vi "5-1 velocità intervento.vi"(2 "stop":bool) -> (0 "delay":u32, 1 "time":u32, 3 "ALARM":bool)   [LabVIEW 2012]
panel:
  # "Realizzare un VI capace di misurare la velocità di intervento di un operatore\n\nValutare il tempo di risposta (Delay) che intercorre tra l'accensione dell'allarme  \ne la pressione del tasto stop e il tempo (Time) di esecuzione del VI."
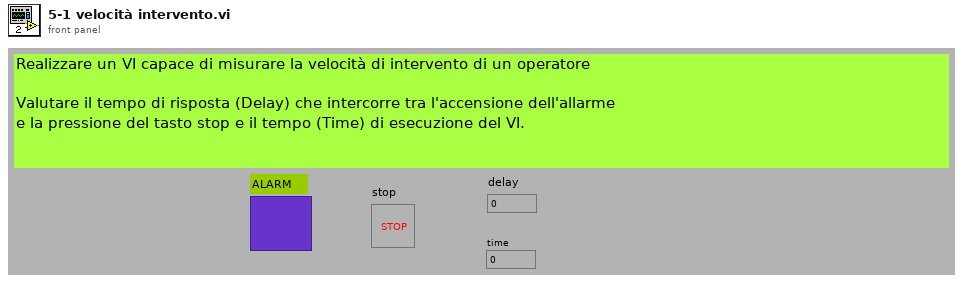
[diagram p1: front panel]
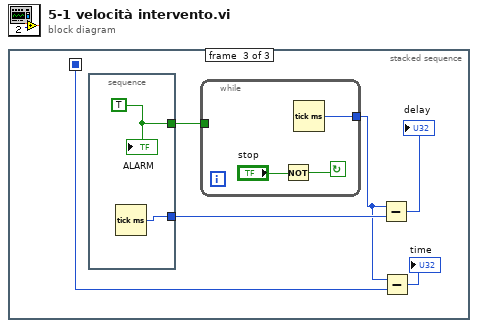
[diagram p0: block diagram]
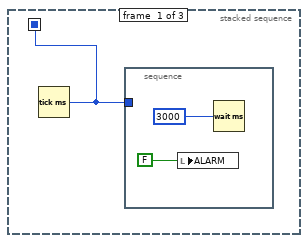
[diagram p2: hidden frame]
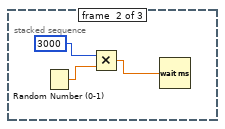
[diagram p3: hidden frame]
diagram:
  n1 = stacked-sequence {
    seq-local: [w1 _ _] -> [_ _ w9]
    frame #0 {
      n2 = Tick Count (ms)() -> (millisecond timer value=w1:u32)
      n3 = stacked-sequence {
        tunnel: w1 -> [_]
        frame #0 {
          n4 = local write "ALARM"(FALSE ("ALARM")) -> ()
          n5 = Wait (ms)(milliseconds to wait=u32 3000) -> ()  [unwired: 1 out]
        }
      }
    }
    frame #1 {
      n6 = Random Number (0-1)() -> (number: 0 to 1=w5:dbl)
      n7 = Multiply(x=3000, y=w5) -> (x*y=w4:dbl)
      n8 = Wait (ms)(milliseconds to wait=w4) -> ()  [unwired: 1 out]
    }
    frame #2 {
      n9 = stacked-sequence {
        tunnel: [w14] -> w11
        tunnel: [w13] -> w8
        frame #0 {
          w14 = TRUE
          n10 = Tick Count (ms)() -> (millisecond timer value=w13:u32)
          "ALARM" <- w14
        }
      }
      n11 = while {
        tunnel: [w17] -> w7
        tunnel: w11 -> [_]
        stop <- w15 continue-if-true
        n12 = Not(x="stop") -> (.not. x?=w15:bool)
        n13 = Tick Count (ms)() -> (millisecond timer value=w17:u32)
      }
      n14 = Subtract(x=w7, y=w8) -> (x-y=→"delay":u32)
      n15 = Subtract(x=w7, y=w9) -> (x-y=→"time":u32)
    }
  }
